vi "Edge Detection_Main Function.vi"(0 "Refnum in":T2, 1 "Process":u16, 2 "Edge Options":T4, 3 "Number of Matches Requested IN":i32, 9 "ROI":T3, 11 "error in (no error)":errorcluster) -> (4 "Image Out":T2, 8 "Edge Information":T1[](array[typedef]) {"Distance (Real-World)" format="%.2f"; "Location (Real-World)"."Y" format="%.2g"; "Location (Real-World)"."X" format="%.2f"; "Noise" format="%.2f"; "Location (Pixel)"."Y" format="%.2g"; "Location (Pixel)"."X" format="%.2f"; "Strength" format="%.2f"; "Distance (Pixel)" format="%.2f"}, 10 "Number of Edges Detected":i32, 15 "error out":errorcluster)   [LabVIEW 2019]
uses:
  <vilib>/vision/Image Controls.llb/IMAQ Image.ctl
  <vilib>/vision/Measure.llb/Edge New.ctl
  <vilib>/vision/NI_Vision_Development_Module.lvlib
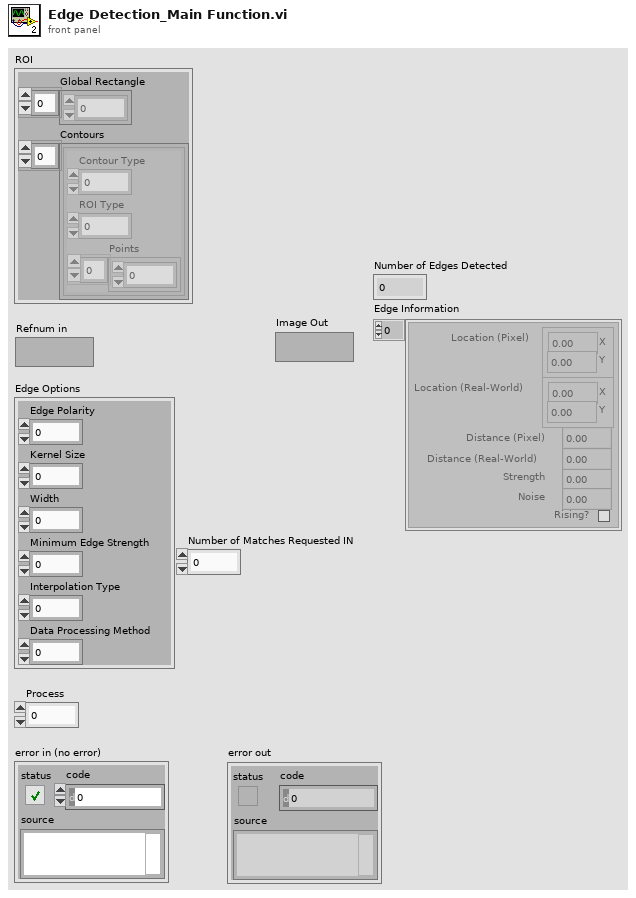
[diagram p1: front panel]
types:
  T1 = typedef "Edge New.ctl" = cluster{"Location (Pixel)":cluster{"X":sgl, "Y":sgl}, "Location (Real-World)":cluster{"X":sgl, "Y":sgl}, "Distance (Pixel)":dbl, "Distance (Real-World)":dbl, "Strength":dbl, "Noise":dbl, "Rising?":bool}
  T2 = typedef "IMAQ Image.ctl" = refnum<image>
  T3 = cluster{"Global Rectangle":i32[], "Contours":cluster{"Contour Type":u32, "ROI Type":u32, "Points":i32[]}[]}
  T4 = cluster{"Edge Polarity":u16, "Kernel Size":u32, "Width":u32, "Minimum Edge Strength":dbl, "Interpolation Type":u16, "Data Processing Method":u16}
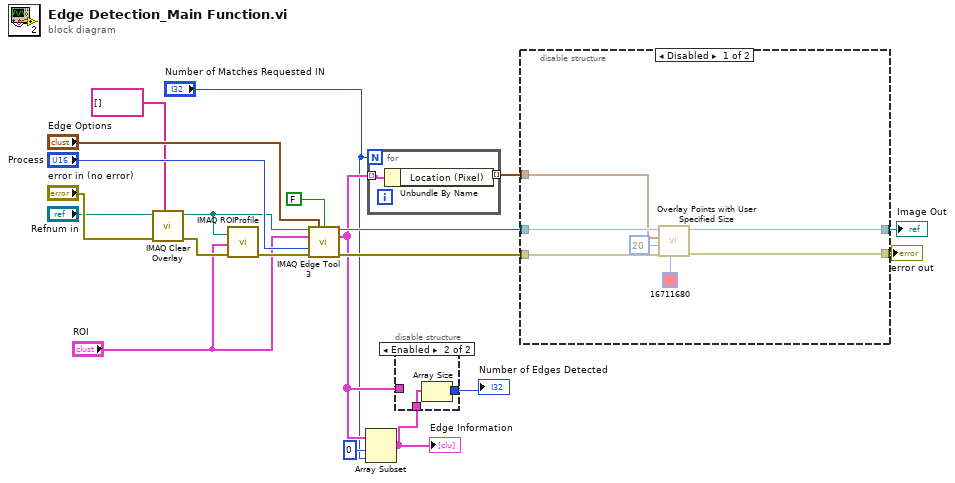
[diagram p0: block diagram]
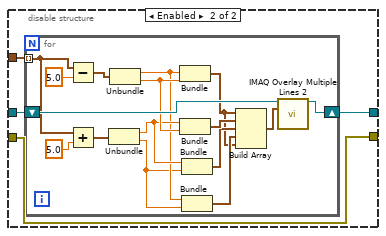
[diagram p2: hidden frame]
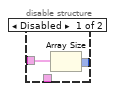
[diagram p3: hidden frame]
diagram:
  n1 = call "IMAQ Clear Overlay"("Groups"=string[] [], "error in (no error)"="error in (no error)", "Image"="Refnum in") -> ("error out"=w12:errorcluster, "Image Out"=w13:T2)  [unwired: 7 in]
  n2 = call "IMAQ ROIProfile"("error in (no error)"=w12, "ROI Descriptor"="ROI", "Image"=w13) -> ("error out"=w16:errorcluster)  [unwired: 1 in, 4 out]
  n3 = call "IMAQ Edge Tool 3"("Image"=w13, "Edge Options"="Edge Options", "Optimized Mode"=FALSE, "ROI Descriptor"="ROI", "Process"="Process", "error in (no error)"=w16) -> ("Image (duplicate)"=w14:T2, "Edge Information"=w2:T1[], "error out"=w15:errorcluster)  [unwired: 5 in, 2 out]
  n4 = Array Subset(array=w2, index=0, length="Number of Matches Requested IN") -> (w4:T1[])
  "Edge Information" <- w4
  n5 = for {
    N: "Number of Matches Requested IN" -> [_]
    tunnel: w2 -> [w22] mode=indexing
    tunnel: [w21] -> w10 mode=indexing
    n6 = Unbundle By Name(w22) -> ("Location (Pixel)"=w21:cluster{"X":sgl, "Y":sgl})
  }
  n7 = disable-structure shown="Enabled" {
    disable-tunnel: w2 -> [w24 _]
    disable-tunnel: w4 -> [_ w26]
    disable-tunnel: [w23 w25] -> w3
    frame Disabled {
      n8 = Array Size(array=w24) -> (size(s)=w23:i32)
    }
    frame Enabled {
      n9 = Array Size(array=w26) -> (size(s)=w25:i32)
    }
  }
  "Number of Edges Detected" <- w3
  n10 = disable-structure shown="Disabled" {
    disable-tunnel: w15 -> [w33 w34]
    disable-tunnel: w14 -> [w32 w36]
    disable-tunnel: w10 -> [w30 w37]
    disable-tunnel: [w29 w34] -> w8
    disable-tunnel: [w28 w35] -> w7
    frame Disabled {
      n11 = call "Overlay Points with User Specified Size.vi"("Color"=u32 16711680, "error in"=w33, "Point Diameter (5)"=u32 20, "Points"=w30, "Image In"=w32) -> ("error out"=w29:errorcluster, "Image Out"=w28:T2)  [unwired: 5 in]
    }
    frame Enabled {
      n12 = for {
        tunnel: w37 -> [w50] mode=indexing
        shift-right: [w38] -> w35
        shift-left: w36 -> [w53]
        n13 = Subtract(x=w50, y=5.0) -> (x-y=w49:cluster{"X":dbl, "Y":dbl})
        n14 = Add(x=w50, y=5.0) -> (x+y=w48:cluster{"X":dbl, "Y":dbl})
        n15 = Unbundle(w48) -> ("X"=w46:dbl, "Y"=w44:dbl)
        n16 = Unbundle(w49) -> ("X"=w45:dbl, "Y"=w47:dbl)
        n17 = Bundle("X"=w45, "Y"=w47) -> (w40:cluster{"X":dbl, "Y":dbl})  [unwired: 1 in]
        n18 = Bundle("X"=w46, "Y"=w47) -> (w43:cluster{"X":dbl, "Y":dbl})  [unwired: 1 in]
        n19 = Bundle("X"=w46, "Y"=w44) -> (w42:cluster{"X":dbl, "Y":dbl})  [unwired: 1 in]
        n20 = Bundle("X"=w45, "Y"=w44) -> (w41:cluster{"X":dbl, "Y":dbl})  [unwired: 1 in]
        n21 = Build Array(w40, w43, w42, w41, w40) -> (w39:cluster{"X":dbl, "Y":dbl}[])
        n22 = call "IMAQ Overlay Multiple Lines 2"("Image"=w53, "Line End Points"=w39) -> ("Image Out"=w38:T2)  [unwired: 12 in, 1 out]
      }
    }
  }
  "error out" <- w8
  "Image Out" <- w7
